vi "LoadMainPanel.vi"(8 "error in (no error)":errorcluster, 11 "Main Class in":refnum<class "Main Class.lvclass">) -> (0 "error out":errorcluster, 2 "This VI":refnum<vi>, 3 "Main Class out":refnum<class "Main Class.lvclass">)   [LabVIEW 2019, in "Main Class.lvclass"]
uses:
  Main Class.lvclass
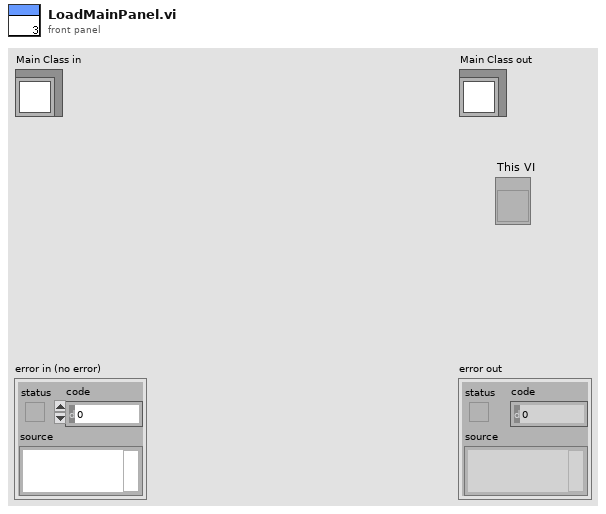
[diagram p1: front panel]
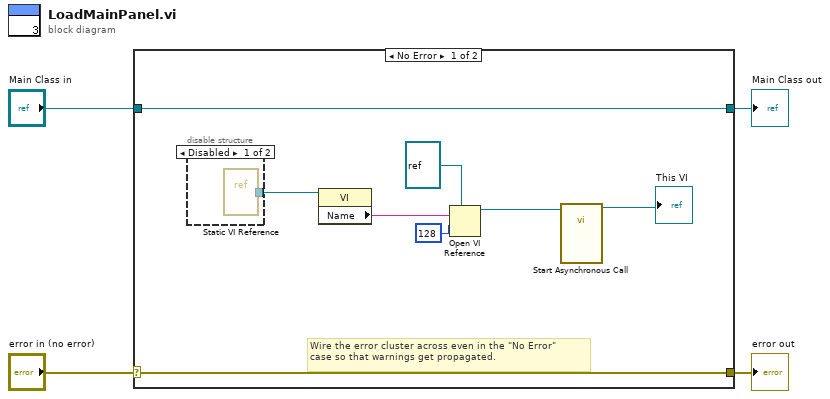
[diagram p0: block diagram]
diagram:
  n1 = case shown="No Error" "error in (no error)" {
    selector: "error in (no error)" -> [w11 w15]
    tunnel: [w11 w15] -> w3
    tunnel: [w12 w14] -> w1
    tunnel: "Main Class in" -> [w12 w14]
    frame No Error {
      # "Wire the error cluster across even in the \"No Error\"\ncase so that warnings get propagated."
      n2 = disable-structure shown="Disabled" {
        disable-tunnel: [w13 _] -> w7
        frame Disabled {
          n3 = vi-ref "Static VI Reference"() -> ("vi reference"=w13:refnum<vi>)
        }
        frame Enabled {
        }
      }
      n4 = property class="VI"(reference=w7) -> ("Name"=w6:string)  [unwired: 1 in, 2 out]
      n5 = Open VI Reference(type specifier VI Refnum (for type only)=refnum<vi> refnum, vi path=w6, options=128) -> (vi reference=w10:refnum<vi>)  [unwired: 3 in, 1 out]
      n6 = call-by-ref "Start Asynchronous Call"(reference=w10) -> (reference out=→"This VI":refnum<vi>)  [unwired: 13 in, 1 out]
    }
    frame Error {
    }
  }
  "error out" <- w3
  "Main Class out" <- w1
